vi "Main.Write Data to VS.vi"(8 "error in":errorcluster, 11 "Data Sessions":T1[](array[typedef]) {"Outgoing.Frames.CountersAndProtections"."Protection Configurations"."CRC Channels"."Data Type" items=["Signed", "Unsigned", "IEEE Float"]; "Trigger.Refs"."Data Reference" format="%.0x"; "Disable.Refs"."Data Reference" format="%.0x"; "Timing.Refs"."Data Reference" format="%.0x"; "Network"."Name" format="%.0x"; "Incoming.Refs"."Data Reference" format="%.0x"; "Outgoing.Refs"."Data Reference" format="%.0x"}) -> (0 "error out":errorcluster, 3 "Data Sessions out":T1[](array[typedef]) {"Outgoing.Frames.CountersAndProtections"."Protection Configurations"."CRC Channels"."Data Type" items=["Signed", "Unsigned", "IEEE Float"]; "Trigger.Refs"."Data Reference" format="%.0x"; "Disable.Refs"."Data Reference" format="%.0x"; "Timing.Refs"."Data Reference" format="%.0x"; "Network"."Name" format="%.0x"; "Incoming.Refs"."Data Reference" format="%.0x"; "Outgoing.Refs"."Data Reference" format="%.0x"})   [LabVIEW 2023, in "J1939 Addon Engine.lvlib"]
uses:
  J1939 Addon Engine.lvlib
  Types/Protocol.XNET Refs.ctl
  Addon Shared/Types/Monitor Settings.ctl
  <vilib>/NI VeriStand/Custom Device API/Block Data Reference.ctl
  <vilib>/NI VeriStand/Custom Device API/Data Reference.ctl
  Types/Main.Outgoing.Frame.Settings.ctl
  Addon Shared/Types/Outgoing Event Trigger Types.ctl
  SubModules/Frame-Protection-Support/Source/Shared/Types/Exported Frame Settings.ctl
  SubModules/Frame-Protection-Support/Source/Shared/Types/Exported Frame Type.ctl
  SubModules/Frame-Protection-Support/Source/Shared/Types/Exported Protection Settings.ctl
  SubModules/Frame-Protection-Support/Source/Shared/Types/Protection Type.ctl
  SubModules/Frame-Protection-Support/Source/Shared/Types/XNET Signal Configuration.ctl
  SubModules/Frame-Protection-Support/Source/Shared/Types/Exported Counter Settings.ctl
  SubModules/Frame-Protection-Support/Source/Shared/Types/Exported Event Trigger Type.ctl
  <vilib>/xnet/xnet.llb/XNET Read (Signal Single-point).vi
  <vilib>/xnet/xnet.llb/XNET Read (Signal XY).vi
  <vilib>/NI VeriStand/Custom Device API/Global Data Refs.vi
  <vilib>/NI VeriStand/Custom Device API/Custom Device API.lvlib
  Addon Shared/J1939 Addon Shared.lvlib
  SubModules/Frame-Protection-Support/Source/Shared/Protection and Counter Support Shared.lvlib
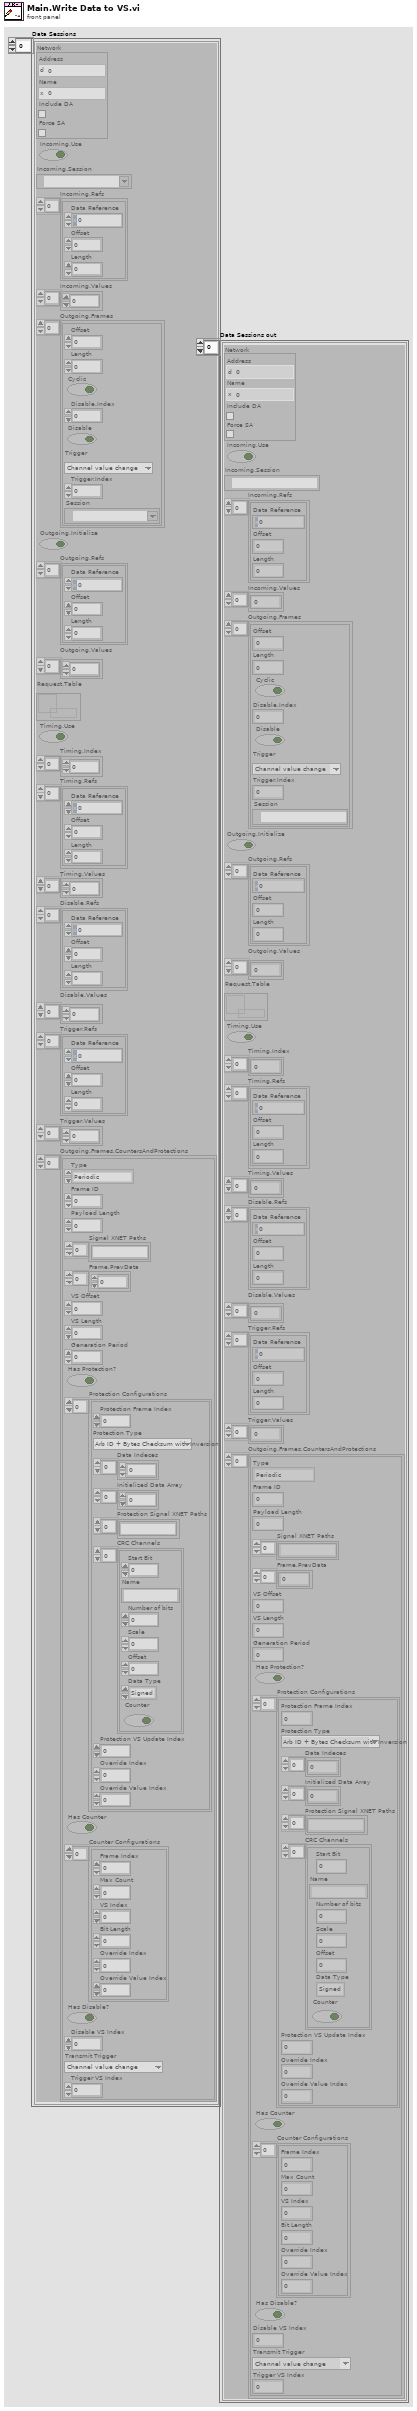
[diagram p1: front panel]
types:
  T1 = typedef "J1939 Addon Engine.lvlib/Protocol.XNET Refs.ctl" = cluster{"Network":T2, "Incoming.Use":bool, "Incoming.Session":refnum<k21>, "Incoming.Refs":T3[], "Incoming.Values":dbl[], "Outgoing.Frames":T5[], "Outgoing.Initialize":bool, "Outgoing.Refs":T3[], "Outgoing.Values":dbl[], "Request.Table":refnum<k33>, "Timing.Use":bool, "Timing.Index":i32[], "Timing.Refs":T3[], "Timing.Values":dbl[], "Disable.Refs":T3[], "Disable.Values":dbl[], "Trigger.Refs":T3[], "Trigger.Values":dbl[], "Outgoing.Frames.CountersAndProtections":T7[]}
  T2 = typedef "J1939 Addon Shared.lvlib/Monitor Settings.ctl" = cluster{"Address":u8, "Name":u64, "Include DA":bool, "Force SA":bool}
  T3 = typedef "Custom Device API.lvlib/Block Data Reference.ctl" = cluster{"Data Reference":T4, "Offset":u64, "Length":u64}
  T4 = typedef "Custom Device API.lvlib/Data Reference.ctl" = i32
  T5 = typedef "J1939 Addon Engine.lvlib/Main.Outgoing.Frame.Settings.ctl" = cluster{"Offset":u32, "Length":u32, "Cyclic":bool, "Disable.Index":i32, "Disable":bool, "Trigger":T6, "Trigger.Index":i32, "Session":refnum<k21>}
  T6 = typedef "J1939 Addon Shared.lvlib/Outgoing Event Trigger Types.ctl" = enum16{"Channel value change", "Trigger channel (not zero)", "Channel value change or trigger channel (not zero)", "Trigger channel (any value change)", "Channel value change or trigger channel (any value change)"}
  T7 = typedef "Protection and Counter Support Shared.lvlib/Exported Frame Settings.ctl" = cluster{"Type":T8, "Frame ID":u32, "Payload Length":u32, "Signal XNET Paths":string[], "Frame.PrevData":dbl[], "VS Offset":i32, "VS Length":i32, "Generation Period":u32, "Has Protection?":bool, "Protection Configurations":T9[], "Has Counter":bool, "Counter Configurations":T12[], "Has Disable?":bool, "Disable VS Index":i32, "Transmit Trigger":T13, "Trigger VS Index":i32}
  T8 = typedef "Protection and Counter Support Shared.lvlib/Exported Frame Type.ctl" = enum16{"Periodic", "Event", "Periodic/Event"}
  T9 = typedef "Protection and Counter Support Shared.lvlib/Exported Protection Settings.ctl" = cluster{"Protection Frame Index":i32, "Protection Type":T10, "Data Indeces":i32[], "Initialized Data Array":dbl[], "Protection Signal XNET Paths":string[], "CRC Channels":T11[], "Protection VS Update Index":i32, "Override Index":i32, "Override Value Index":i32}
  T10 = typedef "Protection and Counter Support Shared.lvlib/Protection Type.ctl" = enum16{"Arb ID + Bytes Checksum with Inversion", "Arb ID + Bytes CRC with Inversion", "Reversed Raw Signal Checksum with Inversion", "Concatenated Two's Compliment"}
  T11 = typedef "Protection and Counter Support Shared.lvlib/XNET Signal Configuration.ctl" = cluster{"Start Bit":i32, "Name":string, "Number of bits":i32, "Scale":dbl, "Offset":dbl, "Data Type":u32, "Counter":bool}
  T12 = typedef "Protection and Counter Support Shared.lvlib/Exported Counter Settings.ctl" = cluster{"Frame Index":i32, "Max Count":dbl, "VS Index":i32, "Bit Length":i64, "Override Index":i32, "Override Value Index":i32}
  T13 = typedef "Protection and Counter Support Shared.lvlib/Exported Event Trigger Type.ctl" = enum16{"Channel value change", "Trigger channel (not zero)", "Channel value change or trigger channel (not zero)", "Trigger channel (any value change)", "Channel value change or trigger channel (any value change)"}
  T14 = cluster{"timestamp":timestamp[], "value":dbl[]}[]
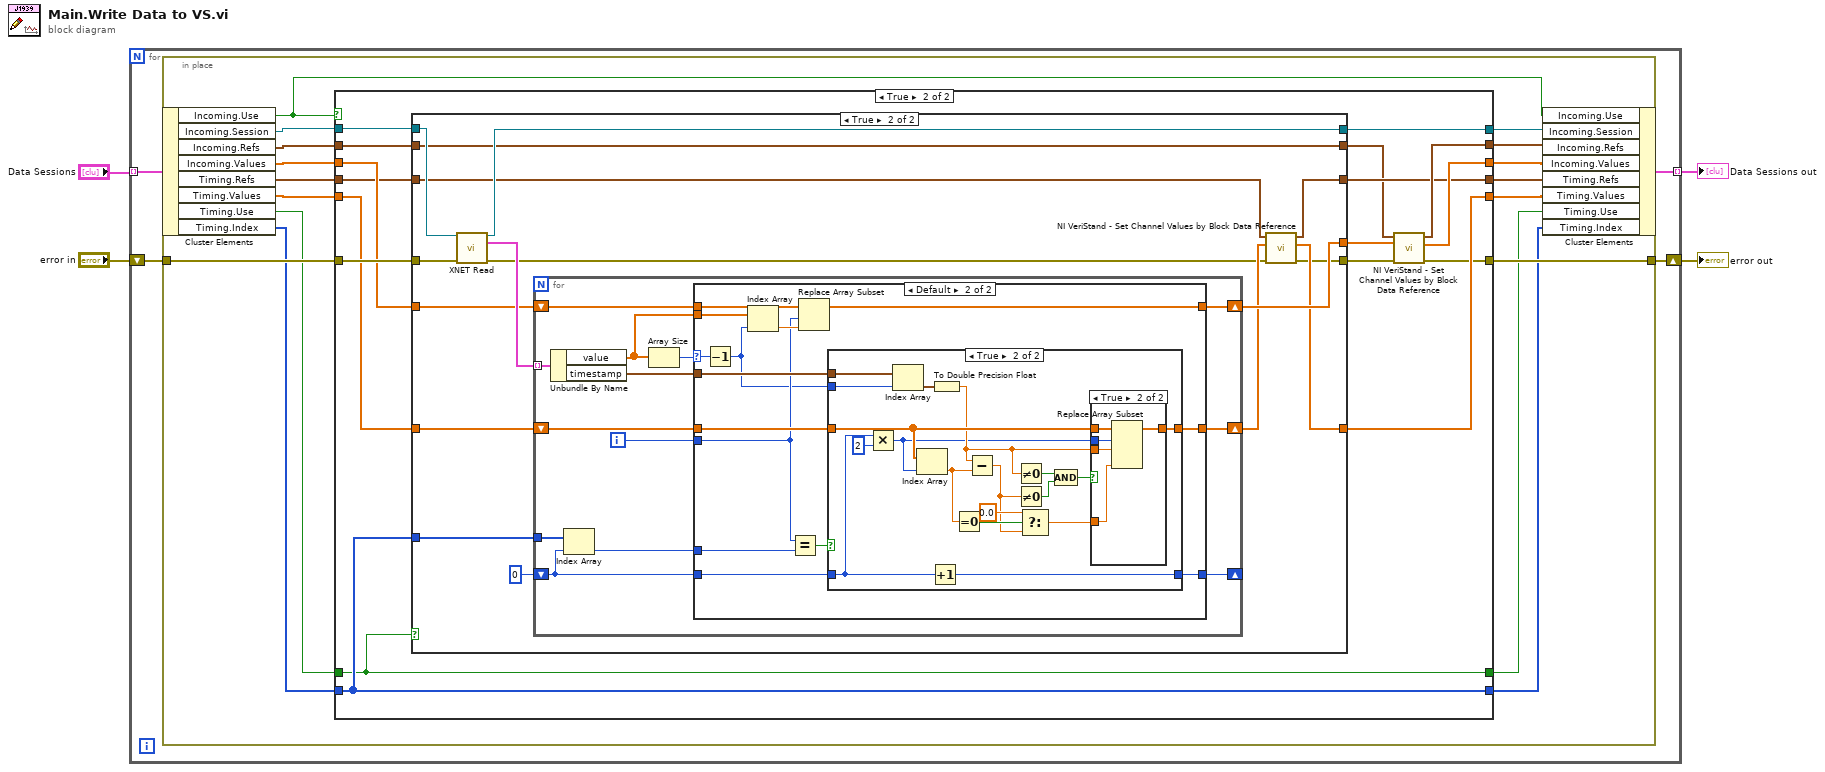
[diagram p0: block diagram]
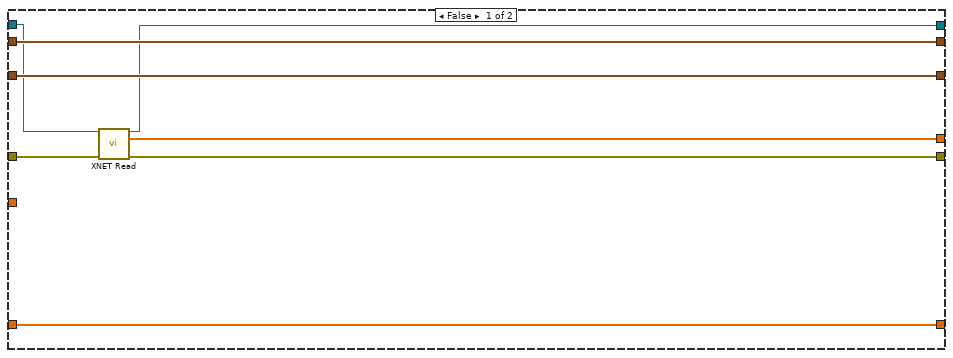
[diagram p3: hidden frame]
diagram:
  n1 = for {
    shift-right: [w7] -> w4
    shift-left: "error in" -> [w8]
    tunnel: "Data Sessions" -> [w6] mode=indexing
    tunnel: [w5] -> w1 mode=indexing
    n2 = in-place {
      in-place-border: w8 -> [w25]
      in-place-border: [w24] -> w7
      n3 = in-place-cluster #1(w6) -> ("Incoming.Use"=w17:bool, "Incoming.Session"=w22:refnum<k21>, "Incoming.Refs"=w21:T3[], "Incoming.Values"=w18:dbl[], "Timing.Refs"=w14:T3[], "Timing.Values"=w16:dbl[], "Timing.Use"=w10:bool, "Timing.Index"=w12:i32[])
      n4 = case shown="True" w17 {
        tunnel: w25 -> [w32 w50]
        tunnel: [w32 w37] -> w24
        tunnel: [w33 w46] -> w23
        tunnel: w22 -> [w30 w49]
        tunnel: w21 -> [w31 w35]
        tunnel: [w30 w48] -> w20
        tunnel: [w31 w47] -> w19
        tunnel: w18 -> [w33 w45]
        tunnel: w16 -> [w29 w43]
        tunnel: [w29 w42] -> w15
        tunnel: w14 -> [w28 w41]
        tunnel: [w28 w40] -> w13
        tunnel: w12 -> [w27 w39]
        tunnel: [w27 w39] -> w11
        tunnel: w10 -> [w26 w34]
        tunnel: [w26 w34] -> w9
        frame False {
        }
        frame True {
          n5 = case shown="True" w34 {
            tunnel: w50 -> [w56 w74]
            tunnel: w49 -> [w55 w73]
            tunnel: [w52 w72] -> w48
            tunnel: w45 -> [_ w70]
            tunnel: [w54 w69] -> w44
            tunnel: w43 -> [w51 w68]
            tunnel: [w51 w66] -> w42
            tunnel: w41 -> [w57 w65]
            tunnel: [w57 w64] -> w40
            tunnel: w39 -> [_ w62]
            tunnel: [w53 w60] -> w38
            tunnel: [w58 w59] -> w36
            tunnel: w35 -> [w58 w59]
            frame False {
              n6 = call-poly <vilib>:"XNET Read.vi"("session in"=w55, "error in (no error)"=w56) -> ("session out"=w52:refnum<k21>, "data"=w54:dbl[], "error out"=w53:errorcluster)  [unwired: 11 in]
            }
            frame True {
              n7 = call-poly <vilib>:"XNET Read.vi"("session in"=w73, "error in (no error)"=w74) -> ("session out"=w72:refnum<k21>, "data"=w71:T14, "error out"=w61:errorcluster)  [unwired: 11 in]
              n8 = for {
                tunnel: w71 -> [w87] mode=indexing
                shift-right: [w85] -> w69
                shift-left: w70 -> [w86]
                shift-right: [w82] -> w67
                shift-left: w68 -> [w83]
                shift-right: [w77] -> _
                shift-left: 0 -> [w80]
                tunnel: w62 -> [w78]
                i -> [w81]
                n9 = Unbundle By Name(w87) -> ("value"=w76:dbl[], "timestamp"=w84:timestamp[])
                n10 = Index Array(array=w78, index=w80) -> (element=w79:i32)
                n11 = Array Size(array=w76) -> (size(s)=w75:i32)
                n12 = case shown="Default" w75 {
                  selector: w75 -> [_ w91]
                  tunnel: w86 -> [w89 w104]
                  tunnel: [w89 w103] -> w85
                  tunnel: w84 -> [_ w101]
                  tunnel: w83 -> [w90 w100]
                  tunnel: [w90 w99] -> w82
                  tunnel: w81 -> [_ w98]
                  tunnel: w80 -> [w88 w97]
                  tunnel: w79 -> [_ w96]
                  tunnel: [w88 w95] -> w77
                  tunnel: w76 -> [_ w93]
                  frame 0 {
                  }
                  frame Default {
                    n13 = Decrement(x=w91) -> (x-1=w92:i32)
                    n14 = Index Array(array=w93, index=w92) -> (element=w102:dbl)
                    n15 = Equal?(x=w98, y=w96) -> (x = y?=w94:bool)
                    n16 = Replace Array Subset(array=w104, new element=w102, index=w98) -> (w103:dbl[])
                    n17 = case shown="True" w94 {
                      tunnel: w101 -> [_ w124]
                      tunnel: w100 -> [w105 w122]
                      tunnel: [w105 w121] -> w99
                      tunnel: w97 -> [w106 w115]
                      tunnel: [w106 w116] -> w95
                      tunnel: w92 -> [_ w107]
                      frame False {
                      }
                      frame True {
                        n18 = Multiply(x=w115, y=2) -> (x*y=w113:i32)
                        n19 = Index Array(array=w124, index=w107) -> (element=w123:timestamp)
                        n20 = Index Array(array=w122, index=w113) -> (element=w112:dbl)
                        n21 = Increment(x=w115) -> (x+1=w116:i32)
                        n22 = To Double Precision Float(number=w123) -> (double precision float=w120:dbl)
                        n23 = Equal To 0?(x=w112) -> (x = 0?=w111:bool)
                        n24 = Subtract(x=w120, y=w112) -> (x-y=w108:dbl)
                        n25 = Not Equal To 0?(x=w120) -> (x != 0?=w119:bool)
                        n26 = Not Equal To 0?(x=w108) -> (x != 0?=w118:bool)
                        n27 = Select(t=0.0, s=w111, f=w108) -> (s? t:f=w109:dbl)
                        n28 = Compound Arithmetic op=AND(w119, w118) -> (w117:bool)
                        n29 = case shown="True" w117 {
                          tunnel: w122 -> [w125 w130]
                          tunnel: w113 -> [_ w129]
                          tunnel: [w125 w128] -> w121
                          tunnel: w109 -> [_ w127]
                          tunnel: w120 -> [_ w126]
                          frame False {
                          }
                          frame True {
                            n30 = Replace Array Subset(array=w130, new element #1=w126, index #1=w129, new element #2=w127) -> (w128:dbl[])  [unwired: 1 in]
                          }
                        }
                      }
                    }
                  }
                }
              }
              n31 = call <vilib>:"NI VeriStand - Set Channel Values by Block Data Reference.vi"("error in (no error)"=w61, "Values Array in"=w67, "Block Data Ref"=w65) -> ("error out"=w60:errorcluster, "Values Array out"=w66:dbl[], "Block Data Ref dup"=w64:T3[])  [unwired: 6 in]
            }
          }
          n32 = call <vilib>:"NI VeriStand - Set Channel Values by Block Data Reference.vi"("error in (no error)"=w38, "Values Array in"=w44, "Block Data Ref"=w36) -> ("error out"=w37:errorcluster, "Values Array out"=w46:dbl[], "Block Data Ref dup"=w47:T3[])  [unwired: 6 in]
        }
      }
      n33 = in-place-cluster #1("Incoming.Use"=w17, "Incoming.Session"=w20, "Incoming.Refs"=w19, "Incoming.Values"=w23, "Timing.Refs"=w13, "Timing.Values"=w15, "Timing.Use"=w9, "Timing.Index"=w11) -> (w5:T1)
    }
  }
  "error out" <- w4
  "Data Sessions out" <- w1
